vi "APUOnLogic.vi"(8 "error in":errorcluster, 11 "UI 1 Data":T1={"System Log"="", "[Array Of Threshold Refs]"=[], "[Array Of Boarder Refs]"=[], "APU Type"="", "APU Setup File"={"Sensor Info"=[], "Variables"=[], "CMM Table 106"=[], "CMM Table 106B "=[], "Accel Config"=[], "Report Sheet 1"=[], "Report Sheet 2"=[], "Report Sheet 3"=[]}, "ActiveValuetoRecordRow"=[], "ReportType"=[], "ReportValue"=[], "ActiveReportSheets"=[], "APUOn"=FALSE, "APUOnTime"=timestamp(0 s since 1904-01-01), "APUOffTime"=timestamp(0 s since 1904-01-01), "Recording"=FALSE, "Test Information"={"APU Part Number:"="555", "Model:"="5", "Serial Number:"="sad", "Customer:"="sad", "Work Order:"="asd", "Pre or Post SB"="Pre SB 49-7711", "Run Count"=0, "APU Selected"="<Select>"}, "APU RUN TIME"=timestamp(0 s since 1904-01-01)} {"APU RUN TIME" format="%<%H:%M:%S>T"; "Test Information"."Run Count" min=0 step=1; "APUOffTime" format="%<%x %.3X>T"; "APUOnTime" format="%<%x %.3X>T"}) -> (0 "error out":errorcluster, 3 "UI 1 Data Out":T1={"System Log"="", "[Array Of Threshold Refs]"=[], "[Array Of Boarder Refs]"=[], "APU Type"="", "APU Setup File"={"Sensor Info"=[], "Variables"=[], "CMM Table 106"=[], "CMM Table 106B "=[], "Accel Config"=[], "Report Sheet 1"=[], "Report Sheet 2"=[], "Report Sheet 3"=[]}, "ActiveValuetoRecordRow"=[], "ReportType"=[], "ReportValue"=[], "ActiveReportSheets"=[], "APUOn"=FALSE, "APUOnTime"=timestamp(0 s since 1904-01-01), "APUOffTime"=timestamp(0 s since 1904-01-01), "Recording"=FALSE, "Test Information"={"APU Part Number:"="555", "Model:"="5", "Serial Number:"="sad", "Customer:"="sad", "Work Order:"="asd", "Pre or Post SB"="Pre SB 49-7711", "Run Count"=0, "APU Selected"="<Select>"}, "APU RUN TIME"=timestamp(0 s since 1904-01-01)} {"APU RUN TIME" format="%<%H:%M:%S>T"; "Test Information"."Run Count" min=0 step=1; "APUOffTime" format="%<%x %.3X>T"; "APUOnTime" format="%<%x %.3X>T"})   [LabVIEW 2018, in "Testing UI 1.lvlib"]
uses:
  Testing UI 1.lvlib
  Private Controls/UI 1 Data.ctl
  Top Level/Shared Controls/APU Setup File.ctl
  File IO/Public Controls/ReportType.ctl
  Controller (Host)/Public Controls/Test Information.ctl
  Controller (Host)/Public VIs/PreorPostSB.ctl
  Controller (Host)/Public Controls/APU Select.ctl
  1089da4a-cd66-4fb8-8968-fb230e91e3d5.vi
  File IO/File IO.lvlib
  Controller (Host)/Controller (Host).lvlib
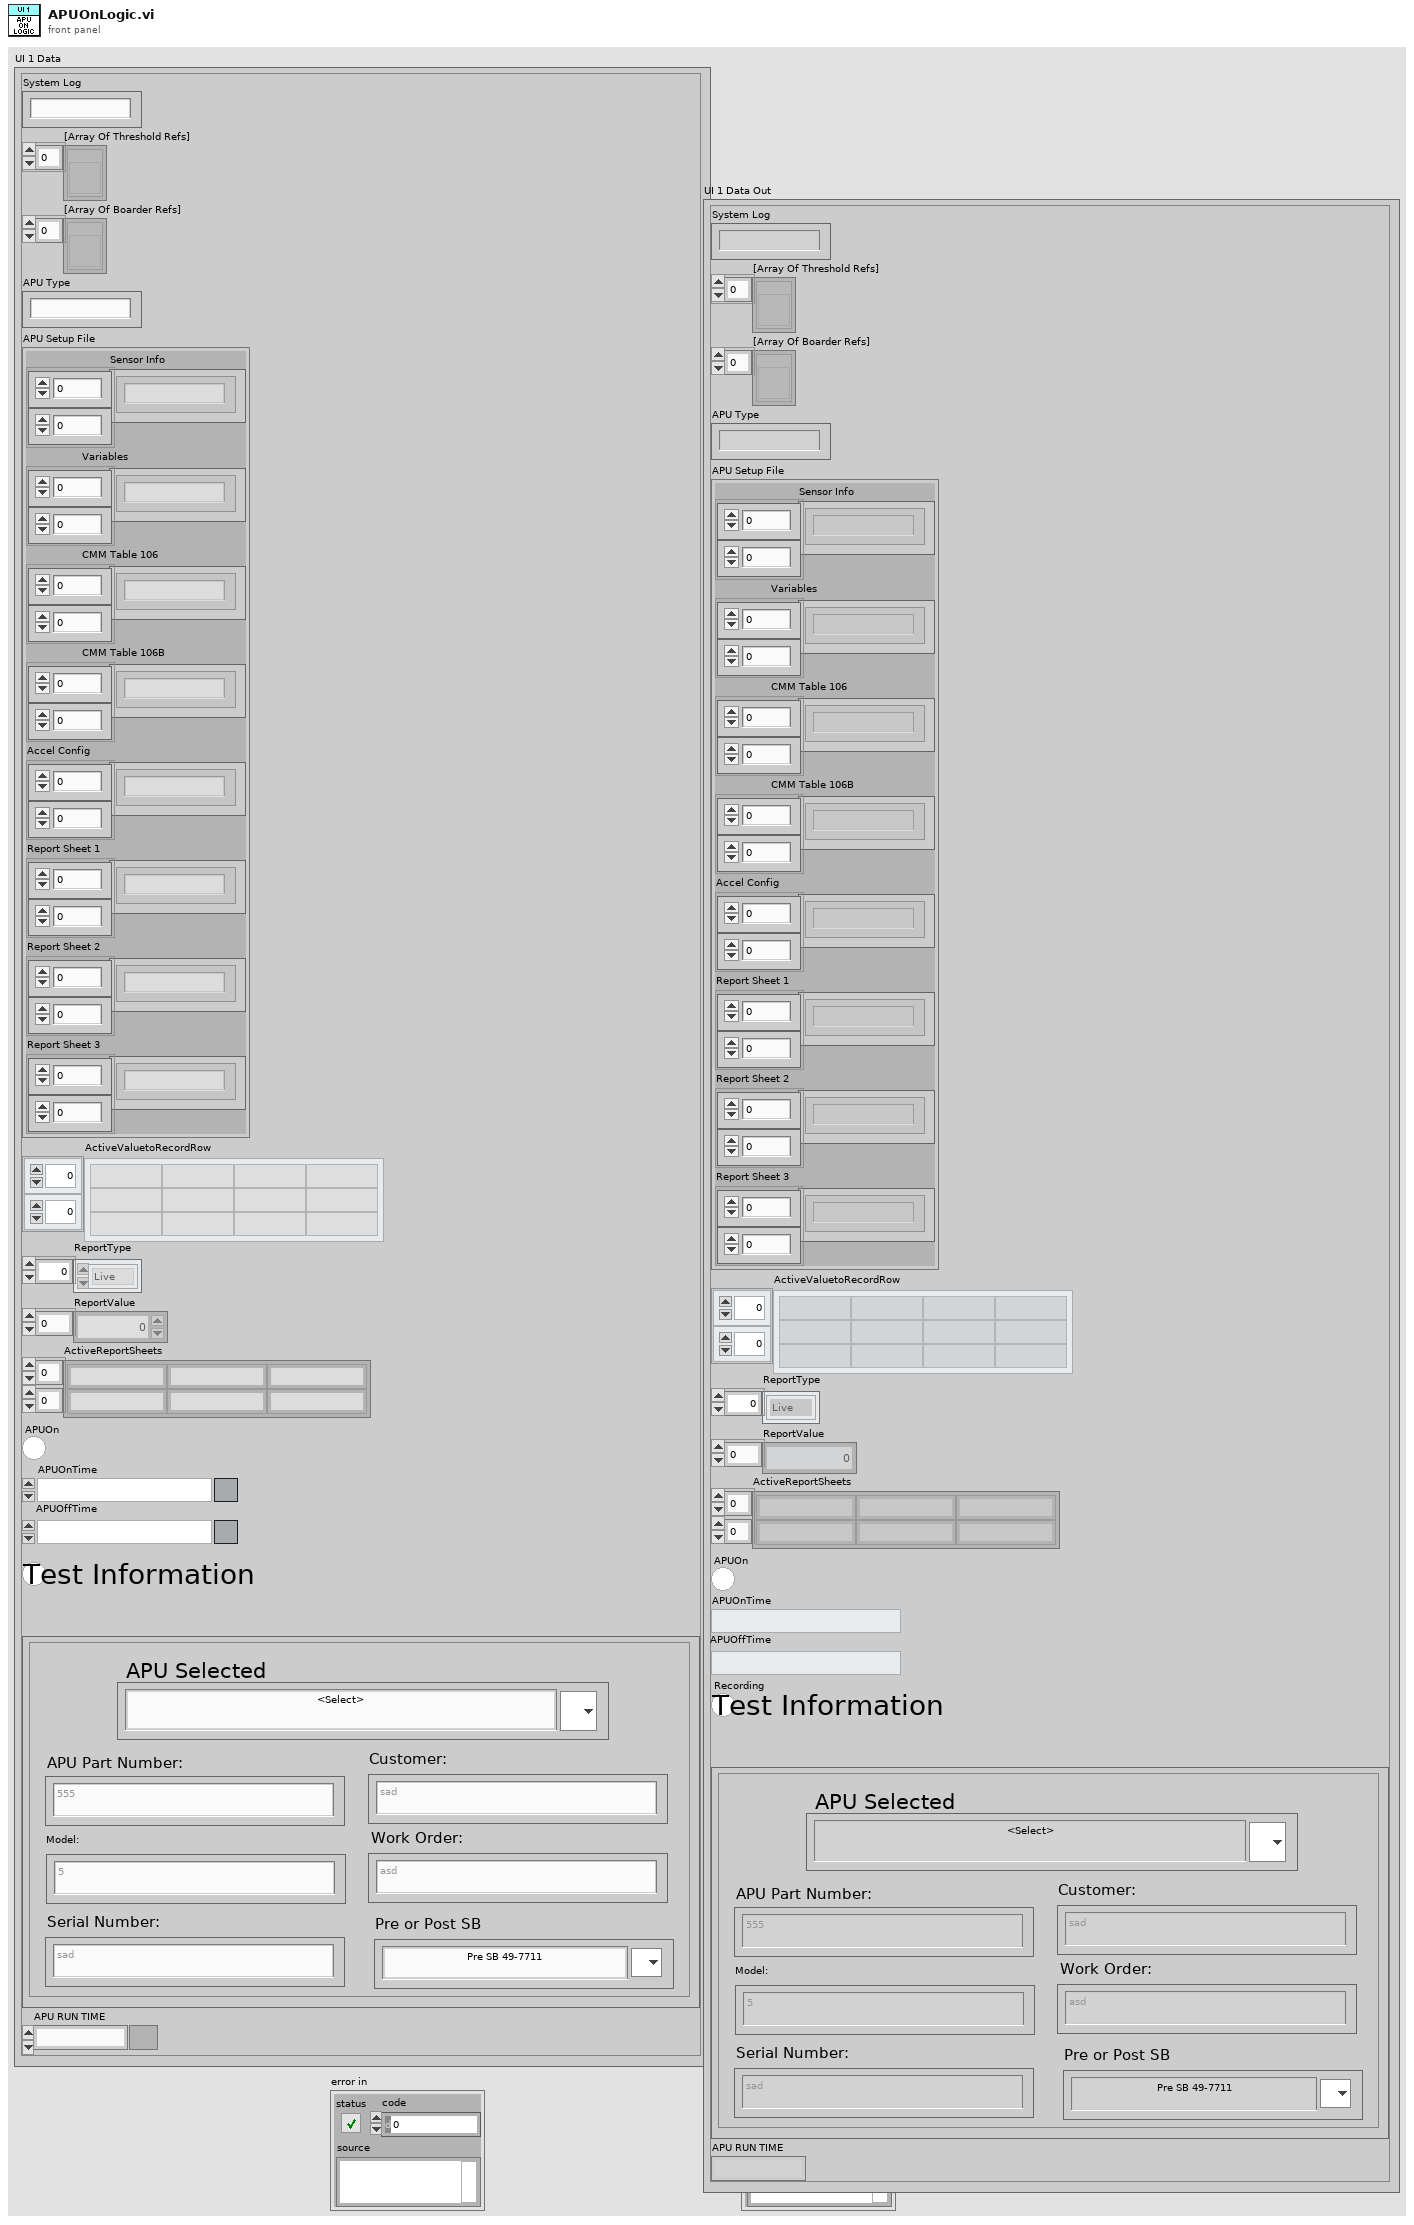
[diagram p1: front panel]
types:
  T1 = typedef "Testing UI 1.lvlib/UI 1 Data.ctl" = cluster{"System Log":string, "[Array Of Threshold Refs]":refnum<vi>[], "[Array Of Boarder Refs]":refnum<vi>[], "APU Type":string, "APU Setup File":T2, "ActiveValuetoRecordRow":string[][], "ReportType":T3[], "ReportValue":dbl[], "ActiveReportSheets":string[][], "APUOn":bool, "APUOnTime":timestamp, "APUOffTime":timestamp, "Recording":bool, "Test Information":T4, "APU RUN TIME":timestamp}
  T2 = typedef "APU Setup File.ctl" = cluster{"Sensor Info":string[][], "Variables":string[][], "CMM Table 106":string[][], "CMM Table 106B ":string[][], "Accel Config":string[][], "Report Sheet 1":string[][], "Report Sheet 2":string[][], "Report Sheet 3":string[][]}
  T3 = typedef "File IO.lvlib/ReportType.ctl" = enum16{"Live", "Min", "Max", "Deviation"}
  T4 = typedef "Controller (Host).lvlib/Test Information.ctl" = cluster{"APU Part Number:":string, "Model:":string, "Serial Number:":string, "Customer:":string, "Work Order:":string, "Pre or Post SB":T5, "Run Count":i32, "APU Selected":T6}
  T5 = typedef "Controller (Host).lvlib/PreorPostSB.ctl" = string
  T6 = typedef "Controller (Host).lvlib/APU Select.ctl" = string
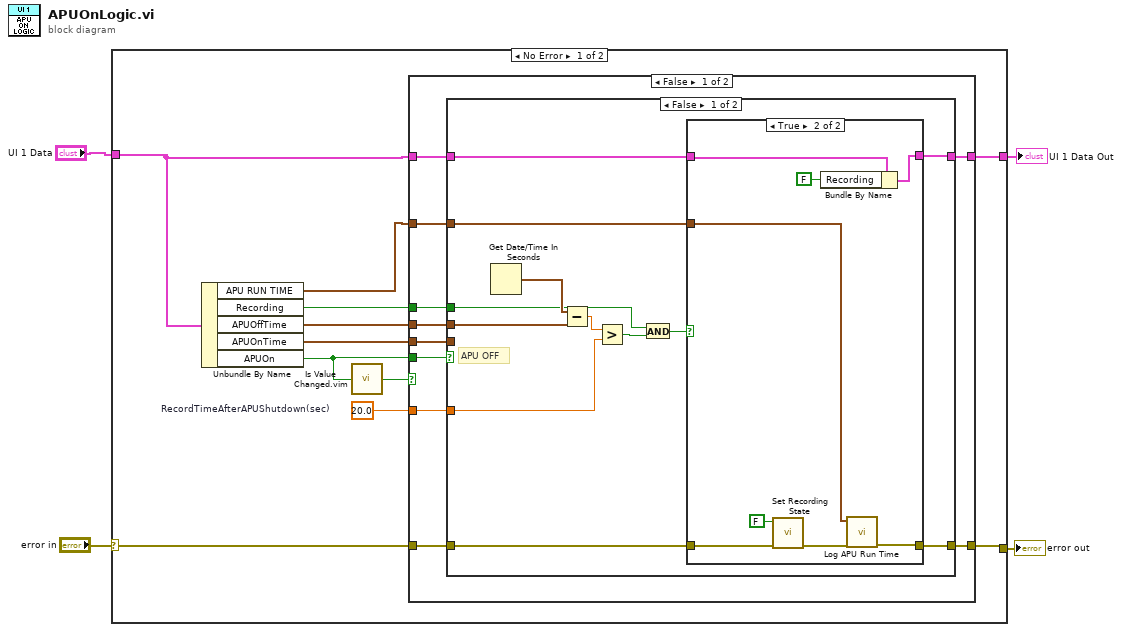
[diagram p0: block diagram]
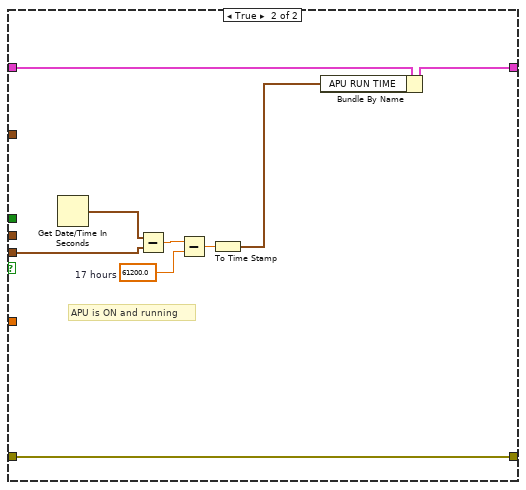
[diagram p3: hidden frame]
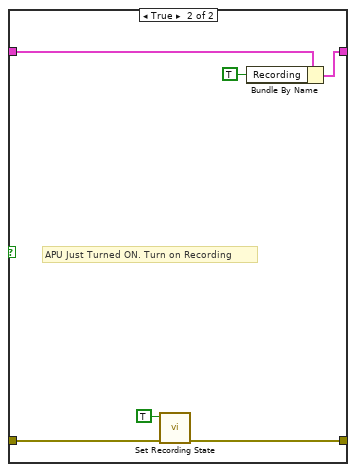
[diagram p5: hidden frame]
diagram:
  n1 = case shown="No Error" "error in" {
    selector: "error in" -> [w12 w71]
    tunnel: [w11 w71] -> w3
    tunnel: "UI 1 Data" -> [w8 w70]
    tunnel: [w7 w70] -> w1
    frame No Error {
      w9 = 20.0  # RecordTimeAfterAPUShutdown(sec)
      n2 = Unbundle By Name(w8) -> ("APU RUN TIME"=w5:timestamp, "Recording"=w6:bool, "APUOffTime"=w10:timestamp, "APUOnTime"=w13:timestamp, "APUOn"=w14:bool)
      n3 = call "Is Value Changed.vim"("value"=w14) -> ("changed or first call?"=w15:bool)
      n4 = case shown="False" w15 {
        tunnel: w14 -> [w25 w61]
        tunnel: w13 -> [w24 _]
        tunnel: w12 -> [w23 w60]
        tunnel: [w22 w59] -> w11
        tunnel: w10 -> [w21 _]
        tunnel: w9 -> [w20 _]
        tunnel: w8 -> [w18 w58]
        tunnel: [w17 w57] -> w7
        tunnel: w6 -> [w19 _]
        tunnel: w5 -> [w16 _]
        frame False {
          n5 = case shown="False" w25 {
            tunnel: w24 -> [_ w52]
            tunnel: [w31 w51] -> w22
            tunnel: w23 -> [w32 w51]
            tunnel: w21 -> [w36 _]
            tunnel: w20 -> [w34 _]
            tunnel: w19 -> [w30 _]
            tunnel: w18 -> [w28 w50]
            tunnel: [w27 w49] -> w17
            tunnel: w16 -> [w26 _]
            frame False {
              # "APU OFF"
              n6 = Get Date/Time In Seconds() -> (seconds since 1Jan1904=w37:timestamp)
              n7 = Subtract(x=w37, y=w36) -> (x-y=w35:dbl)
              n8 = Greater?(x=w35, y=w34) -> (0:w29:bool)
              n9 = And(x=w30, y=w29) -> (x .and. y?=w33:bool)
              n10 = case shown="True" w33 {
                tunnel: w32 -> [w39 w47]
                tunnel: [w39 w40] -> w31
                tunnel: w28 -> [w38 w45]
                tunnel: [w38 w44] -> w27
                tunnel: w26 -> [_ w42]
                frame False {
                  # "Recording is either off or the time\nhas not been reached yet."
                }
                frame True {
                  n11 = call "Set Recording State.vi"("error in (no error)"=w47, "Recording State"=FALSE) -> ("error out"=w41:errorcluster)  [unwired: 9 in]
                  n12 = Bundle By Name(cluster=w45, "Recording"=FALSE) -> (w44:T1)
                  n13 = call "Log APU Run Time.vi"("error in (no error)"=w41, "APU RUN TIME"=w42) -> ("error out"=w40:errorcluster)  [unwired: 9 in]
                }
              }
            }
            frame True {
              w55 = 61200.0  # 17 hours
              # "APU is ON and running"
              n14 = Get Date/Time In Seconds() -> (seconds since 1Jan1904=w56:timestamp)
              n15 = Subtract(x=w56, y=w52) -> (x-y=w54:dbl)
              n16 = Subtract(x=w54, y=w55) -> (x-y=w53:dbl)
              n17 = To Time Stamp(1:w53) -> (0:w48:timestamp)
              n18 = Bundle By Name(cluster=w50, "APU RUN TIME"=w48) -> (w49:T1)
            }
          }
        }
        frame True {
          n19 = case shown="False" w61 {
            tunnel: w60 -> [w63 w69]
            tunnel: [w63 w68] -> w59
            tunnel: w58 -> [w62 w66]
            tunnel: [w62 w65] -> w57
            frame False {
              # "APU Just Turned OFF. We are still Recording.\nRecord while the APU spins down."
            }
            frame True {
              # "APU Just Turned ON. Turn on Recording"
              n20 = call "Set Recording State.vi"("error in (no error)"=w69, "Recording State"=TRUE) -> ("error out"=w68:errorcluster)  [unwired: 9 in]
              n21 = Bundle By Name(cluster=w66, "Recording"=TRUE) -> (w65:T1)
            }
          }
        }
      }
    }
    frame Error {
    }
  }
  "error out" <- w3
  "UI 1 Data Out" <- w1
